vi "Encode error.vi"(6 "First decimal to code":u8=5, 8 "error in (no error)":errorcluster, 11 "Data in":dbl[](array[numeric]) format="%#_15g") -> (3 "Error tagged data out":dbl[](array[numeric]) format="%#_15g")   [LabVIEW 2019]
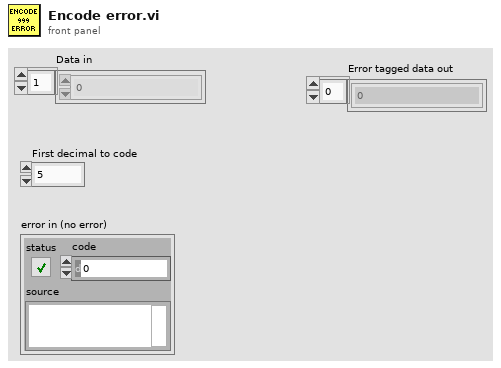
[diagram p1: front panel]
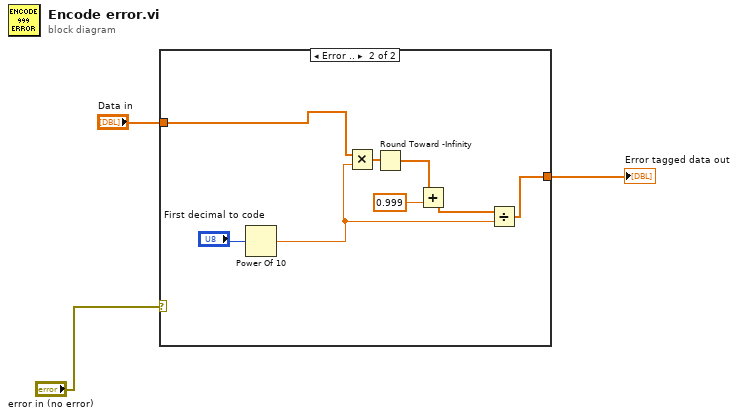
[diagram p0: block diagram]
diagram:
  n1 = case shown="Error .." "error in (no error)" {
    tunnel: "Data in" -> [w4 w6]
    tunnel: [w4 w5] -> w2
    frame No Error {
    }
    frame Error {
      n2 = Power Of 10(x="First decimal to code") -> (10^x=w7:dbl)
      n3 = Multiply(x=w6, y=w7) -> (x*y=w12:dbl[])
      n4 = Round Toward -Infinity(1:w12) -> (0:w11:dbl[])
      n5 = Add(x=w11, y=0.999) -> (x+y=w10:dbl[])
      n6 = Divide(x=w10, y=w7) -> (x/y=w5:dbl[])
    }
  }
  "Error tagged data out" <- w2
